vi "Start Sync.vi"(8 "error in (no error)":errorcluster, 10 "current time":timestamp, 11 "gRPC Server in":refnum<class "HVC7.lvclass">) -> (0 "error out":errorcluster, 3 "gRPC Server out":refnum<class "HVC7.lvclass">)   [LabVIEW 2019, in "HVC7.lvlib" / "HVC7.lvclass"]
uses:
  HVC7.lvclass
  HVC7.lvclass/HVC7.ctl
  RPC Messages/measurementservice_QueryResponse/measurementservice_QueryResponse_Data.ctl
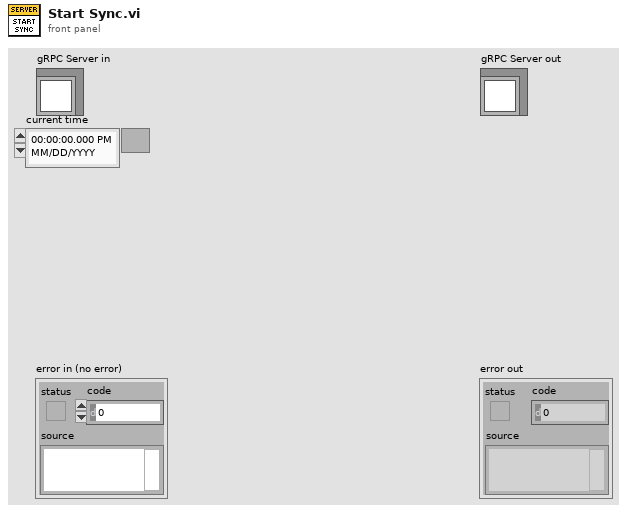
[diagram p1: front panel]
types:
  T1 = typedef "HVC7.lvlib/HVC7.lvclass/measurementservice_QueryResponse_Data.ctl" = cluster{"message":string, "status":i32}
  T2 = typedef "HVC7.lvlib/HVC7.lvclass/Server gRPC UEs.ctl" = cluster{"Invoke gRPC UE":refnum<user-event>, "Query gRPC UE":refnum<user-event>, "Register gRPC UE":refnum<user-event>, "OpenDIOSession gRPC UE":refnum<user-event>, "ReadDI gRPC UE":refnum<user-event>, "WriteDO gRPC UE":refnum<user-event>, "CloseDIOSession gRPC UE":refnum<user-event>}
  T3 = typedef "HVC7.lvlib/gprc-lvsupport.lvlib/grpcId.ctl" = u64
  T4 = typedef "HVC7.lvlib/HVC7.lvclass/measurementservice_QueryRequest_Data.ctl" = cluster{"query":string}
  T5 = typedef "HVC7.lvlib/HVC7.lvclass/measurementservice_DIOOpenSessionRequest_Data.ctl" = cluster{"DIOSessionName":string, "DIOlines":string}
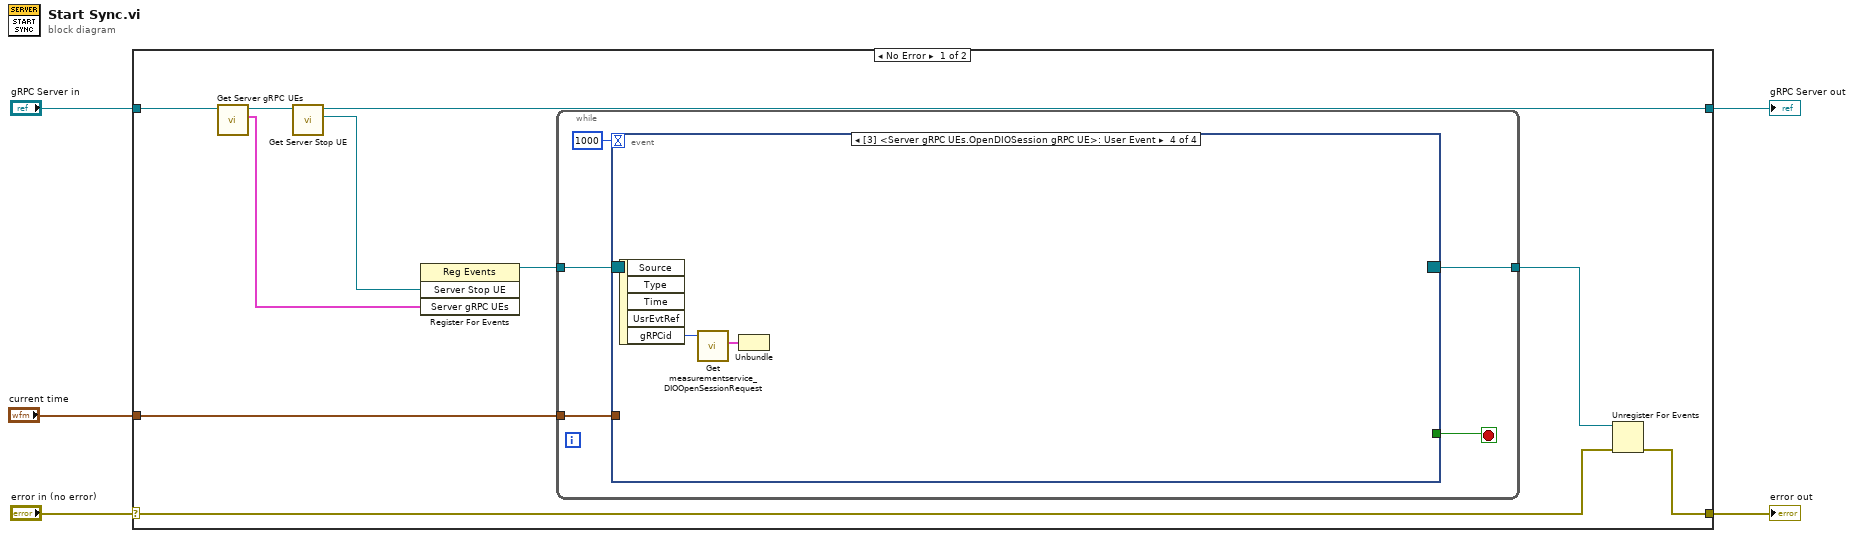
[diagram p0: block diagram]
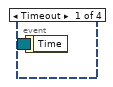
[diagram p2: hidden frame]
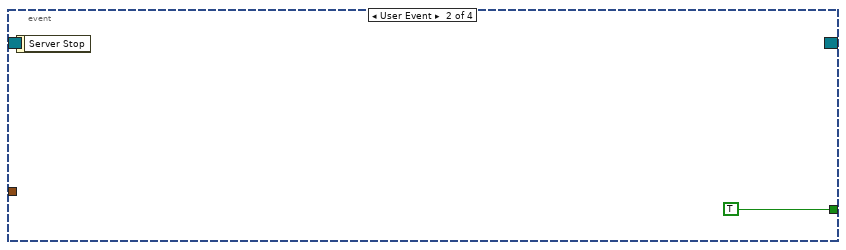
[diagram p3: hidden frame]
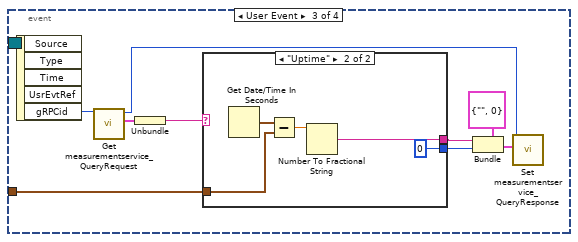
[diagram p4: hidden frame]
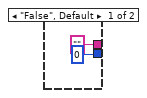
[diagram p5: hidden frame]
diagram:
  n1 = case shown="No Error" "error in (no error)" {
    selector: "error in (no error)" -> [w8 w41]
    tunnel: [w7 w41] -> w4
    tunnel: [w11 w40] -> w2
    tunnel: "gRPC Server in" -> [w15 w40]
    tunnel: "current time" -> [w6 _]
    frame No Error {
      n2 = call "Get Server gRPC UEs.vi"("OOP Server in"=w15) -> ("Server gRPC UEs"=w12:T2, "OOP Server out"=w14:refnum<class "HVC7.lvclass">)  [unwired: 9 in]
      n3 = call "Get Server Stop UE.vi"("OOP Server in"=w14) -> ("Server Stop UE"=w13:refnum<user-event>, "OOP Server out"=w11:refnum<class "HVC7.lvclass">)  [unwired: 9 in]
      n4 = register-events(w13, w12) -> (reference out=w10:refnum<event-registration>)  [unwired: 2 in, 1 out]
      n5 = while {
        tunnel: w10 -> [w20]
        tunnel: [w18] -> w9
        tunnel: w6 -> [w16]
        stop <- w19 stop-if-true
        n6 = event "RPC Methods Event Structure" shown="[3] <Server gRPC UEs.OpenDIOSession gRPC UE>: User Event" {
          selector: w20 -> [_ _ _ _]
          dyn-events: [_ _ _ _] -> w18
          timeout: 1000 -> [_ _ _ _]
          tunnel: [_ TRUE _ _] -> w19
          tunnel: w16 -> [_ _ w27 _]
          event Timeout {
            n7 = event-data() -> ()  [unwired: 1 in, 1 out]
          }
          event User Event {
            n8 = event-data() -> ()  [unwired: 1 in, 1 out]
          }
          event User Event {
            n9 = event-data() -> ("gRPCid"=w30:T3)  [unwired: 1 in, 4 out]
            n10 = call "Get measurementservice_QueryRequest.vi"("gRPCid"=w30) -> ("Message Data"=w29:T4, "gRPCid out"=w22:T3)  [unwired: 8 in, 1 out]
            n11 = Unbundle(w29) -> ("query"=w28:string)
            n12 = case shown="\"Uptime\"" w28 {
              tunnel: w27 -> [_ w36]
              tunnel: [0 ("status") 0 ("status")] -> w24
              tunnel: ["" w33] -> w23
              frame "False", Default {
              }
              frame "Uptime" {
                n13 = Get Date/Time In Seconds() -> (seconds since 1Jan1904=w37:timestamp)
                n14 = Subtract(x=w37, y=w36) -> (x-y=w35:dbl)
                n15 = Number To Fractional String(number=w35) -> (F-format string=w33:string)  [unwired: 3 in]
              }
            }
            n16 = Bundle(cluster=T1 {"message"="", "status"=0} ("Message Data"), "message"=w23, "status"=w24) -> (w25:T1)
            n17 = call "Set measurementservice_QueryResponse.vi"("Message Data"=w25, "gRPCid"=w22) -> ()  [unwired: 9 in, 1 out]
          }
          event User Event {
            n18 = event-data() -> ("gRPCid"=w39:T3)  [unwired: 1 in, 4 out]
            n19 = call "Get measurementservice_DIOOpenSessionRequest.vi"("gRPCid"=w39) -> ("Message Data"=w38:T5)  [unwired: 8 in, 2 out]
            n20 = Unbundle(w38) -> ()  [unwired: 2 out]
          }
        }
      }
      n21 = Unregister For Events(event registration refnum=w9, error in=w8) -> (error out=w7:errorcluster)
    }
    frame Error {
    }
  }
  "error out" <- w4
  "gRPC Server out" <- w2
